vi "Timeout Tracker.vi"(10 "Mouse Not Moving?":bool, 11 "Timeout SP":dbl caption="Timeout" format="%.1f") -> (2 "Timeout Timer":dbl, 3 "Timeout":bool)   [LabVIEW 2018]
panel:
  # "secs"
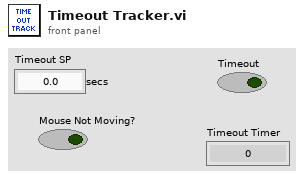
[diagram p1: front panel]
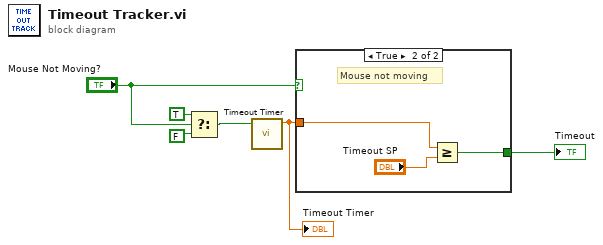
[diagram p0: block diagram]
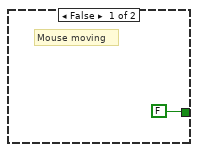
[diagram p2: hidden frame]
diagram:
  n1 = Select(t=TRUE ("Enabled"), s="Mouse Not Moving?", f=FALSE ("Enabled")) -> (s? t:f=w2:bool)
  n2 = call "Timeout Timer.vi"("Enabled"=w2) -> ("Time Into Trial (secs)"=w1:dbl)  [unwired: 10 in]
  "Timeout Timer" <- w1
  n3 = case shown="True" "Mouse Not Moving?" {
    tunnel: [FALSE w10] -> w6
    tunnel: w1 -> [_ w8]
    frame False {
      # "Mouse moving"
    }
    frame True {
      # "Mouse not moving"
      n4 = Greater Or Equal?(x=w8, y="Timeout SP") -> (x >= y?=w10:bool)
    }
  }
  "Timeout" <- w6
